vi "Read Parameter FIFO.vi"(8 "Error In":errorcluster, 11 "Parameters in":T1) -> (0 "Error Out":errorcluster, 3 "Parameters out":T1)   [LabVIEW 2014, in "Waveform-Processing-Custom-Device Engine.lvlib"]
uses:
  Waveform-Processing-Custom-Device Engine.lvlib
  Types/Async Parameters.ctl
  Types/Async FIFOs.ctl
  <vilib>/NI Veristand/Custom Device Waveform API/Single Waveform Read (DBL)/Single Waveform Read (DBL).lvclass
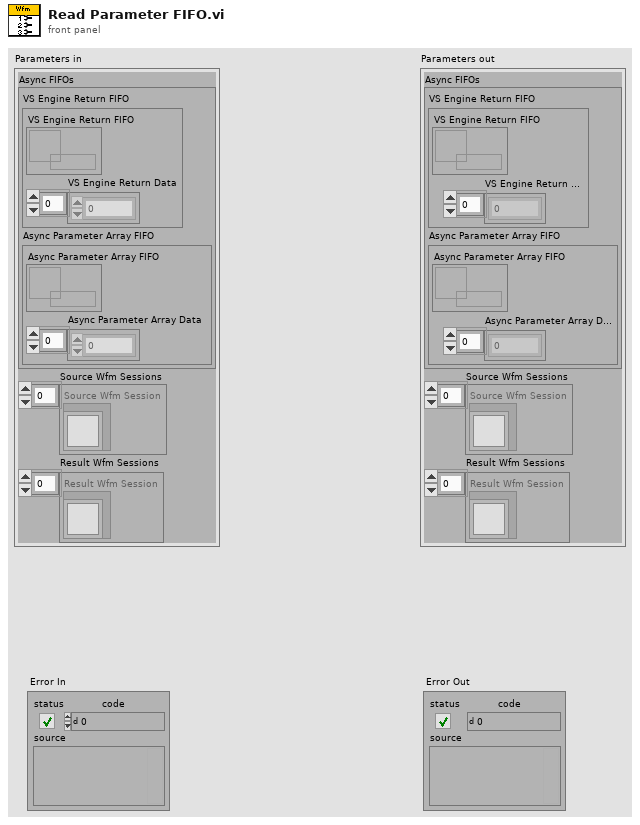
[diagram p1: front panel]
types:
  T1 = typedef "Waveform-Processing-Custom-Device Engine.lvlib/Async Parameters.ctl" = cluster{"Async FIFOs":T2, "Source Wfm Sessions":refnum<class "Single Waveform Read (DBL).lvclass">[], "Result Wfm Sessions":refnum<class "Single Waveform Read (DBL).lvclass">[]}
  T2 = typedef "Waveform-Processing-Custom-Device Engine.lvlib/Async FIFOs.ctl" = cluster{"VS Engine Return FIFO":cluster{"VS Engine Return FIFO":refnum<k33>, "VS Engine Return Data":dbl[]}, "Async Parameter Array FIFO":cluster{"Async Parameter Array FIFO":refnum<k33>, "Async Parameter Array Data":dbl[]}}
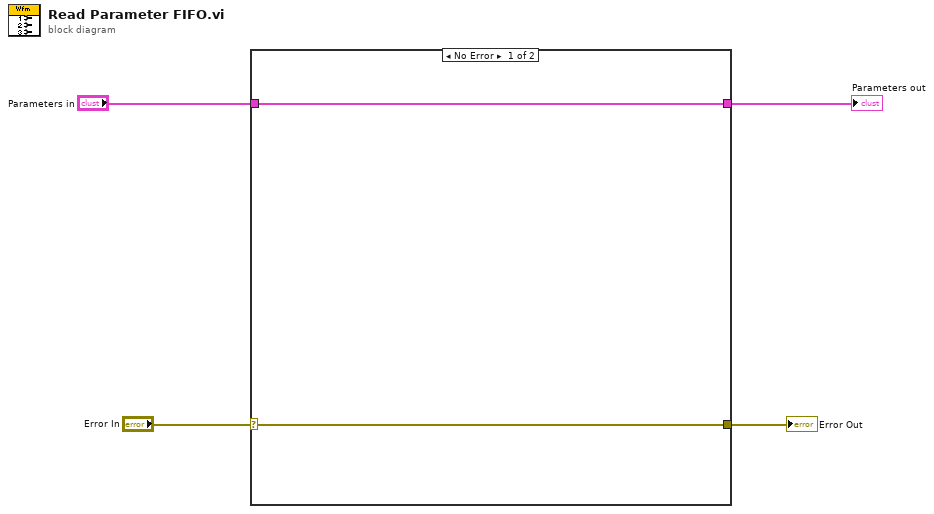
[diagram p0: block diagram]
diagram:
  n1 = case shown="No Error" "Error In" {
    selector: "Error In" -> [w5 w8]
    tunnel: [w5 w8] -> w3
    tunnel: "Parameters in" -> [w6 w7]
    tunnel: [w6 w7] -> w1
    frame No Error {
    }
    frame Error {
    }
  }
  "Error Out" <- w3
  "Parameters out" <- w1
